vi "CustomErrors_DDS.vi"(8 "error in (no error)":errorcluster) -> (0 "error out":errorcluster)   [LabVIEW 2013]
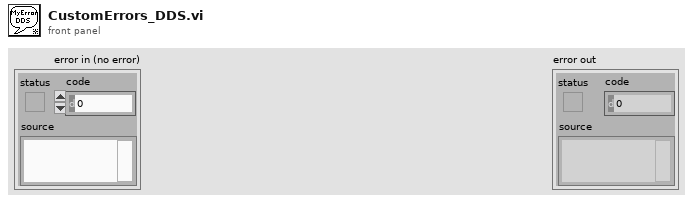
[diagram p1: front panel]
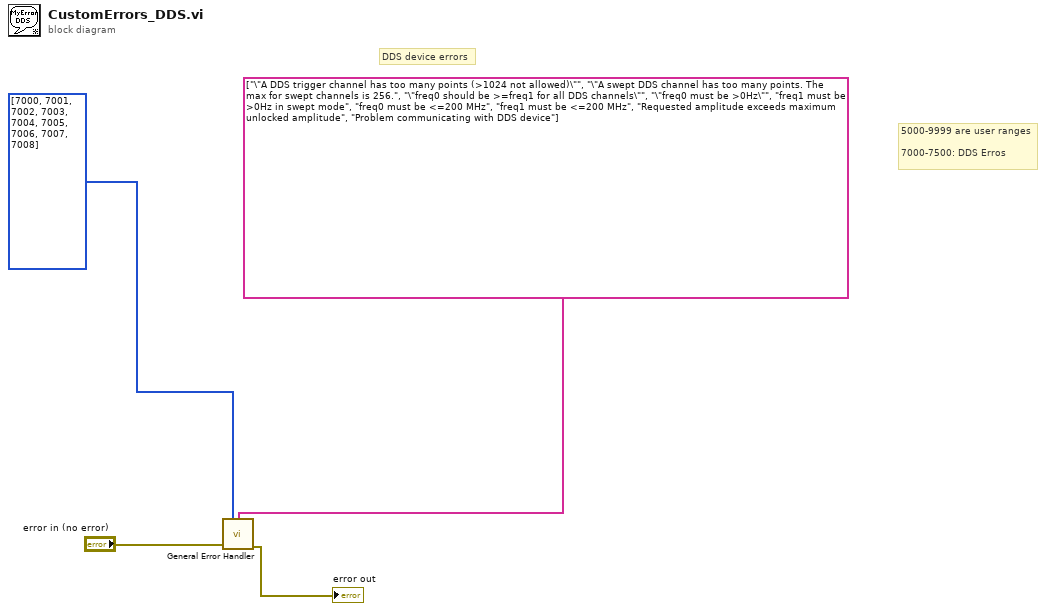
[diagram p0: block diagram]
diagram:
  # "DDS device errors"
  # "5000-9999 are user ranges\n\n7000-7500: DDS Erros"
  n1 = call <vilib>:"General Error Handler.vi"("[user-defined codes]"=i32[] [7000, 7001, 7002, 7003, 7004, 7005, 7006, 7007, 7008], "[user-defined descriptions]"=string[] ["\"A DDS trigger channel has too many points (>1024 not allowed)\"", "\"A swept DDS channel has too many points. The max for swept channels is 256.", "\"freq0 should be >=freq1 for all DDS channels\"", "\"freq0 must be >0Hz\"", "freq1 must be >0Hz in swept mode", "freq0 must be <=200 MHz", "freq1 must be <=200 MHz", "Requested amplitude exceeds maximum unlocked amplitude", "Problem communicating with DDS device"], "error in (no error)"="error in (no error)") -> ("error out"=→"error out":errorcluster)  [unwired: 8 in, 4 out]
